vi "lfieldpanel_DO_set_experiment.vi"(8 "error in (no error)":errorcluster, 10 "experiment_name":string, 11 "lightfield_panel in":refnum<class "lightfield_panel.lvclass">) -> (0 "error out":errorcluster, 3 "lightfield_panel out":refnum<class "lightfield_panel.lvclass">)   [LabVIEW 2015, in "lightfield_panel.lvclass"]
uses:
  lightfield_panel.lvclass
  lightfield/lightfield_class.lvclass
  UI/panel_class/panel.lvclass
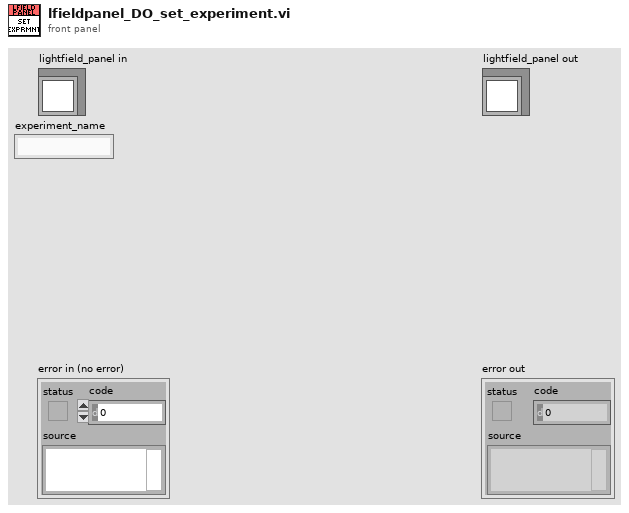
[diagram p1: front panel]
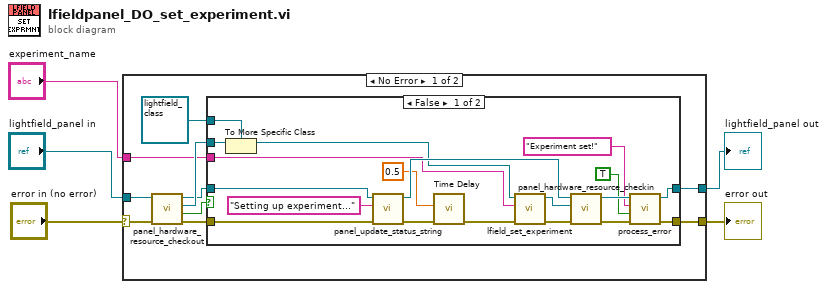
[diagram p0: block diagram]
diagram:
  n1 = case shown="No Error" "error in (no error)" {
    selector: "error in (no error)" -> [w14 w38]
    tunnel: [w8 w38] -> w4
    tunnel: [w7 w37] -> w2
    tunnel: "lightfield_panel in" -> [w15 w37]
    tunnel: "experiment_name" -> [w6 _]
    frame No Error {
      n2 = call "panel_hardware_resource_checkout.vi"("error in (no error)"=w14, "panel in"=w15) -> ("error out"=w10:errorcluster, "timed out?"=w13:bool, "hardware.lvclass"=w11:refnum<class "hardware.lvclass">, "panel out"=w9:refnum<class "lightfield_panel.lvclass">)  [unwired: 6 in]
      n3 = case shown="False" w13 {
        tunnel: refnum<class "lightfield_class.lvclass"> refnum ("lightfield_class.lvclass") -> [w34 _]
        tunnel: w11 -> [w33 _]
        tunnel: w10 -> [w26 w35]
        tunnel: w9 -> [w25 w36]
        tunnel: [w30 w35] -> w8
        tunnel: [w29 w36] -> w7
        tunnel: w6 -> [w19 _]
        frame False {
          n4 = To More Specific Class(target class=w34, reference=w33) -> (specific class reference=w22:refnum<class "lightfield_class.lvclass">)  [unwired: 1 in, 1 out]
          n5 = call-dynamic "panel_update_status_string.vi"("error in (no error)"=w26, "String"="Setting up experiment...", "lightfield_panel in"=w25) -> ("error out"=w17:errorcluster, "lightfield_panel out"=w24:refnum<class "lightfield_panel.lvclass">)  [unwired: 7 in]
          n6 = call "Time Delay"("error in (no error)"=w17, "Delay Time (s)"=0.5) -> ("error out"=w16:errorcluster)  [unwired: 9 in]
          n7 = call "lfield_set_experiment.vi"("error in (no error)"=w16, "experiment_name"=w19, "lightfield_class in"=w22) -> ("error out"=w20:errorcluster, "lightfield_class out"=w21:refnum<class "lightfield_class.lvclass">)  [unwired: 7 in]
          n8 = call "panel_hardware_resource_checkin.vi"("error in (no error)"=w20, "hardware.lvclass"=w21, "panel in"=w24) -> ("error out"=w31:errorcluster, "panel out"=w32:refnum<class "lightfield_panel.lvclass">)  [unwired: 7 in]
          n9 = call "process_error.vi"("error in (no error)"=w31, "Update Status"=TRUE, "No Error Message"="Experiment set!", "lightfield_panel in"=w32) -> ("error out"=w30:errorcluster, "lightfield_panel out"=w29:refnum<class "lightfield_panel.lvclass">)  [unwired: 6 in]
        }
        frame True {
        }
      }
    }
    frame Error {
    }
  }
  "error out" <- w4
  "lightfield_panel out" <- w2
